vi "RunTest.vi"(8 "error in (no error)":errorcluster, 11 "reference in":refnum<class "Test_Template.lvclass">) -> (0 "error out":errorcluster, 1 "State":T1, 3 "reference in":refnum<class "Test_Template.lvclass">)   [LabVIEW 2017]
uses:
  Test_Template.lvclass
  Components/TestView_Base.lvlibp/TestView_Base.lvclass
  Components/MES_Base.lvlibp/MES_Base.lvclass
  TestView_Bailey/TestsState.ctl
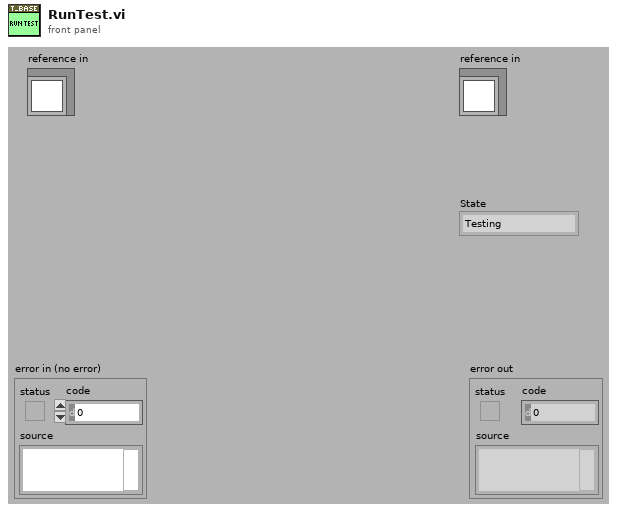
[diagram p1: front panel]
types:
  T1 = typedef "TestsState.ctl" = enum16{"Testing", "Pass", "Fail", "Abort", "Fault"}
  T2 = typedef "Test_Template.lvlib/Test_Template.lvclass/ObjectAttributes.ctl" = cluster{"Config":T3}
  T3 = typedef "Test_Template.lvlib/Test_Template.lvclass/Config.ctl" = cluster{"default":string}
  T4 = cluster{"Code":string, "Name":string, "Description":string, "Group":string, "IsGroup":bool, "Tag":string, "Method":string, "Parrameter":string, "DataType":enum16{"NA", "String", "Boolean", "Int", "Dbl"}, "Value":variant, "Status":enum16{"Pending", "Pass", "Fail"}, "LimitLo":variant, "LimitHi":variant, "StringMatch":string, "BooleanMatch":bool, "DisplayFormat":string, "Units":string, "TestTime":dbl}
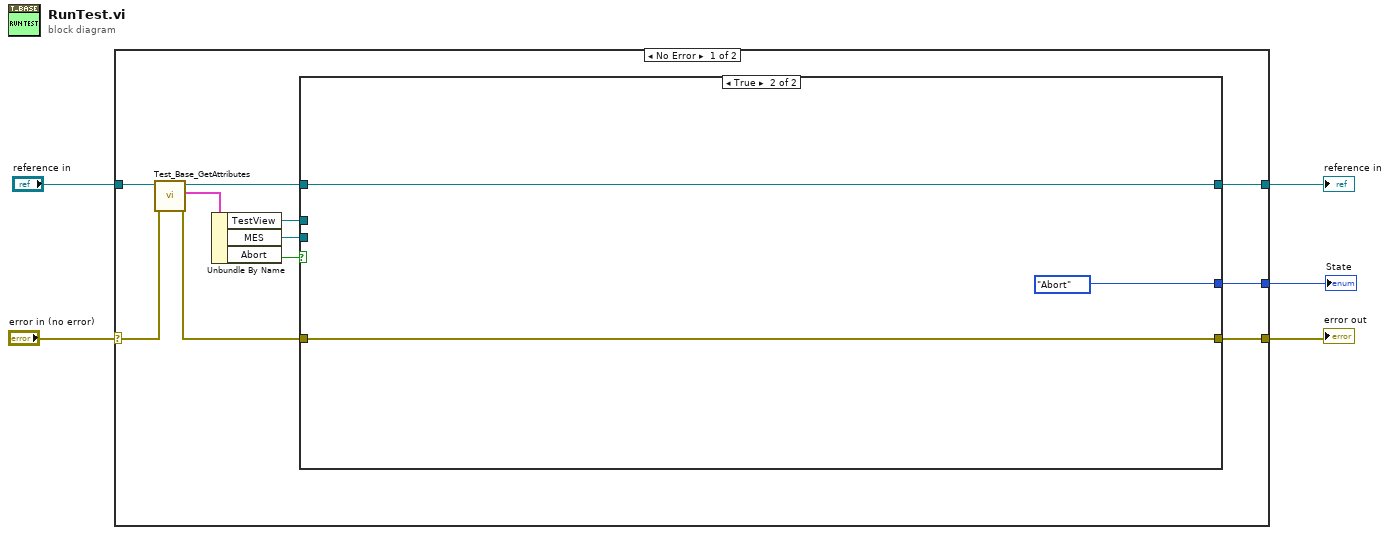
[diagram p0: block diagram]
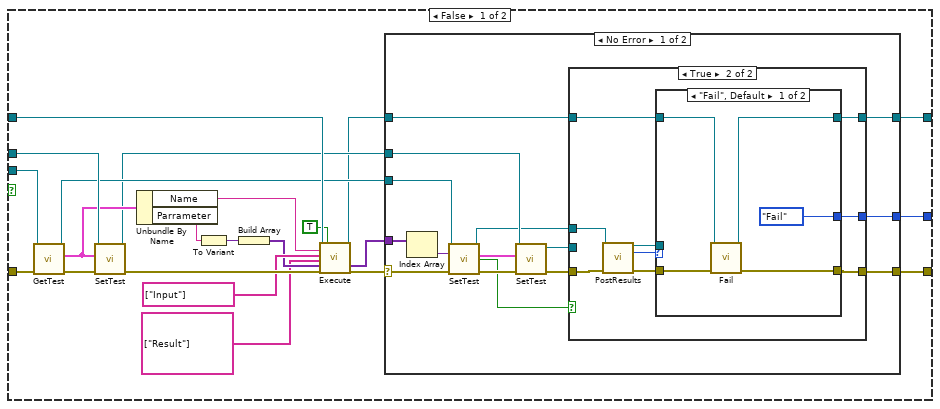
[diagram p2: hidden frame]
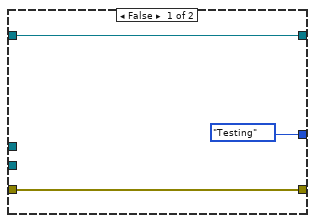
[diagram p3: hidden frame]
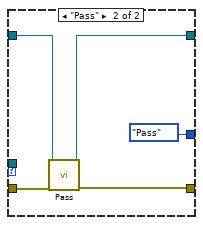
[diagram p4: hidden frame]
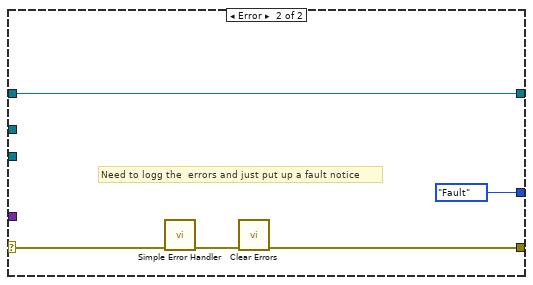
[diagram p5: hidden frame]
diagram:
  n1 = case shown="No Error" "error in (no error)" {
    selector: "error in (no error)" -> [w16 w85]
    tunnel: [w8 w85] -> w4
    tunnel: [w9 w84] -> w2
    tunnel: "reference in" -> [w14 w84]
    tunnel: [w6 _] -> w1
    frame No Error {
      n2 = call "Test_Base_GetAttributes.vi"("error in (no error)"=w16, "reference in"=w14) -> ("error out"=w13:errorcluster, "Data"=w15:T2, "reference out"=w10:refnum<class "Test_Template.lvclass">)  [unwired: 6 in, 1 out]
      n3 = Unbundle By Name(w15) -> ("TestView"=w11:refnum<class "TestView_Base.lvclass">, "MES"=w12:refnum<class "MES_Base.lvclass">, "Abort"=w7:bool)
      n4 = case shown="True" w7 {
        tunnel: w13 -> [w38 w82]
        tunnel: w12 -> [w36 _]
        tunnel: w11 -> [w35 _]
        tunnel: w10 -> [w33 w83]
        tunnel: [w20 w83] -> w9
        tunnel: [w19 w82] -> w8
        tunnel: [w17 TestsState."Abort" ("State")] -> w6
        frame False {
          n5 = call-dynamic "GetTest.vi"("error in (no error)"=w38, "reference in"=w36) -> ("error out"=w37:errorcluster, "Test"=w32:T4, "reference in"=w23:refnum<class "MES_Base.lvclass">)  [unwired: 7 in]
          n6 = call-dynamic "SetTest.vi"("error in (no error)"=w37, "Test"=w32, "reference in"=w35) -> ("error out"=w34:errorcluster, "reference in"=w22:refnum<class "TestView_Base.lvclass">)  [unwired: 7 in]
          n7 = Unbundle By Name(w32) -> ("Name"=w31:string, "Parrameter"=w28:string)
          n8 = To Variant(anything=w28) -> (Variant=w27:variant)
          n9 = Build Array(w27) -> (w26:variant[])
          n10 = call-dynamic "Execute.vi"("reference in"=w33, "cmd"=w31, "controls"=string[] ["Input"], "indicators"=string[] ["Result"] ("controls"), "control data"=w26, "error in (no error)"=w34, "must_exist"=TRUE) -> ("reference out"=w21:refnum<class "Test_Template.lvclass">, "indicator data"=w24:variant[], "error out"=w18:errorcluster)  [unwired: 8 in, 2 out]
          n11 = case shown="No Error" w18 {
            selector: w18 -> [w40 w78]
            tunnel: w24 -> [w53 _]
            tunnel: w23 -> [w52 _]
            tunnel: w22 -> [w49 _]
            tunnel: w21 -> [w43 w79]
            tunnel: [w42 w79] -> w20
            tunnel: [w41 w76] -> w19
            tunnel: [w39 TestsState."Fault" ("State")] -> w17
            frame No Error {
              n12 = Index Array(array=w53) -> (element=w51:variant)  [unwired: 1 in]
              n13 = call-dynamic "SetTest.vi"("reference in"=w52, "Value"=w51, "error in (no error)"=w40) -> ("reference in"=w44:refnum<class "MES_Base.lvclass">, "Test"=w48:T4, "Complete"=w45:bool, "error out"=w50:errorcluster)  [unwired: 8 in, 1 out]
              n14 = call-dynamic "SetTest.vi"("error in (no error)"=w50, "Test"=w48, "reference in"=w49) -> ("error out"=w47:errorcluster, "reference in"=w46:refnum<class "TestView_Base.lvclass">)  [unwired: 7 in]
              n15 = case shown="True" w45 {
                tunnel: w47 -> [w55 w65]
                tunnel: w46 -> [_ _]
                tunnel: w44 -> [_ w64]
                tunnel: w43 -> [w56 w60]
                tunnel: [w56 w59] -> w42
                tunnel: [w55 w58] -> w41
                tunnel: [TestsState."Testing" ("State") w57] -> w39
                frame False {
                }
                frame True {
                  n16 = call-dynamic "PostResults.vi"("reference in"=w64, "error in (no error)"=w65) -> ("reference in"=w61:refnum<class "MES_Base.lvclass">, "Result"=w62:enum16{"Pending", "Pass", "Fail"}, "error out"=w63:errorcluster)  [unwired: 11 in]
                  n17 = case shown="\"Fail\", Default" w62 {
                    tunnel: w63 -> [w68 w75]
                    tunnel: w61 -> [_ _]
                    tunnel: w60 -> [w70 w74]
                    tunnel: [w69 w73] -> w59
                    tunnel: [w67 w72] -> w58
                    tunnel: [TestsState."Fail" ("State") TestsState."Pass" ("State")] -> w57
                    frame "Fail", Default {
                      n18 = call-dynamic "Fail.vi"("error in (no error)"=w68, "reference in"=w70) -> ("error out"=w67:errorcluster, "reference in"=w69:refnum<class "Test_Template.lvclass">)  [unwired: 8 in]
                    }
                    frame "Pass" {
                      n19 = call-dynamic "Pass.vi"("error in (no error)"=w75, "reference in"=w74) -> ("error out"=w72:errorcluster, "reference in"=w73:refnum<class "Test_Template.lvclass">)  [unwired: 8 in]
                    }
                  }
                }
              }
            }
            frame Error {
              # "Need to logg the\t errors and just put up a fault notice"
              n20 = call <vilib>:"Simple Error Handler.vi"("error in (no error)"=w78) -> ("error out"=w77:errorcluster)  [unwired: 4 in, 4 out]
              n21 = call <vilib>:"Clear Errors.vi"("error in (no error)"=w77) -> ("error out"=w76:errorcluster)  [unwired: 5 in, 1 out]
            }
          }
        }
        frame True {
        }
      }
    }
    frame Error {
    }
  }
  "error out" <- w4
  "reference in" <- w2
  "State" <- w1
